vi "AlazarCreateStreamFile.vi"(2 "error in (no error)":errorcluster, 3 "File Path":string, 4 "Handle":u64) -> (0 "error out":errorcluster, 1 "Handle":u64)   [LabVIEW 2018]
doc: "Create a binary data file for this board, and enable saving AutoDMA data from this board to disk."
panel:
  out "Error Code":u32
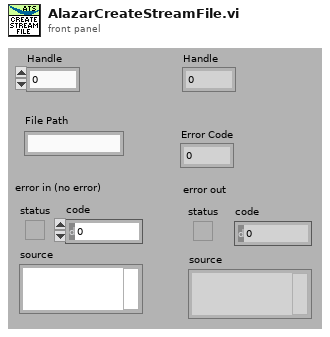
[diagram p1: front panel]
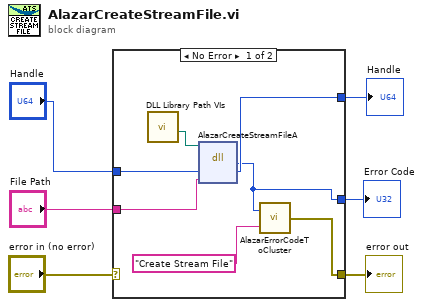
[diagram p0: block diagram]
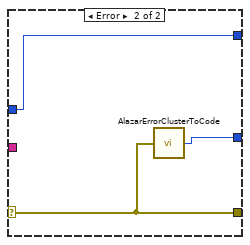
[diagram p2: hidden frame]
diagram:
  n1 = case shown="No Error" "error in (no error)" {
    selector: "error in (no error)" -> [_ w16]
    tunnel: [w11 w16] -> w5
    tunnel: "Handle" -> [w13 w15]
    tunnel: [w12 w15] -> w3
    tunnel: "File Path" -> [w10 _]
    tunnel: [w9 w14] -> w1
    frame No Error {
      n2 = call "DLL Library Path VIs.vi"() -> ("Alazar"=w7:path)  [unwired: 9 in, 2 out]
      n3 = dll-call lib="C:/Project/SerialSectOCT - FFT GPU/SerialSectOCT/Labview Software/DLL/ATSApi.dll" fn="AlazarCreateStreamFileA"(path in=w7, "handle"=w13, "filePath"=w10) -> ("return type"=w9:u32, "handle"=w12:u64)  [unwired: 3 in, 2 out]
      n4 = call "AlazarErrorCodeToCluster.vi"("Message"="Create Stream File", "Error Code"=w9) -> ("error out"=w11:errorcluster)
    }
    frame Error {
      n5 = call "AlazarErrorClusterToCode.vi"("error in (no error)"=w16) -> ("Error Code"=w14:u32)
    }
  }
  "Handle" <- w3
  "error out" <- w5
  "Error Code" <- w1
